vi "Square Root - RM.vi"(1 "Real Matrix A":T2) -> (0 "sqrt(A)":T1)   [LabVIEW 2020, in "NI_Matrix.lvlib"]
doc: "Computes the square root of the input matrix."
uses:
  <vilib>/Analysis/Matrix/NI_Matrix.lvlib
  <vilib>/Analysis/Matrix/Datatypes/RealMatrix.ctl
  <vilib>/Analysis/Matrix/Datatypes/ComplexMatrix.ctl
  <vilib>/Analysis/7linalg.llb/Real Matrix Square Root.vi
  <vilib>/Analysis/NI_AALBase.lvlib
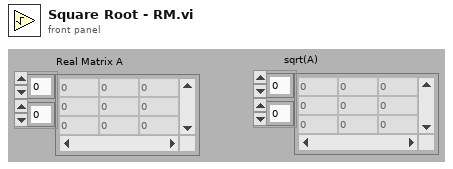
[diagram p1: front panel]
types:
  T1 = typedef "NI_Matrix.lvlib/ComplexMatrix.ctl" = cdb[][]
  T2 = typedef "NI_Matrix.lvlib/RealMatrix.ctl" = dbl[][]
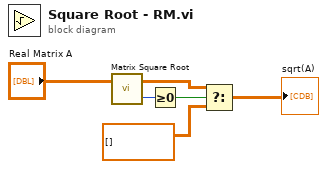
[diagram p0: block diagram]
diagram:
  n1 = call-poly <vilib>:"Matrix Square Root.vi"("Input Matrix"="Real Matrix A") -> ("error"=w1:i32, "Matrix Square Root"=w2:T1)  [unwired: 1 in]
  n2 = Greater Or Equal To 0?(x=w1) -> (x >= 0?=w6:bool)
  n3 = Select(t=w2, s=w6, f=T1 [] ("sqrt(A)")) -> (s? t:f=→"sqrt(A)":T1)
